vi "Push Incons.vi"(10 "node ref in":refnum<data-value>, 11 "adstar in":refnum<class "NI_Robotics_AnytimeDStar.lvclass">) -> (2 "node ref out":refnum<data-value>, 3 "adstar out":refnum<class "NI_Robotics_AnytimeDStar.lvclass">)   [LabVIEW 2017, in "NI_Robotics_AnytimeDStar.lvclass"]
uses:
  <vilib>/robotics/Navigation/Anytime D Star/NI_Robotics_AnytimeDStar.lvclass
  <vilib>/robotics/Navigation/shared/MapNode/AbstractDstarNode/NI_Robotics_AbstractDstarNode.lvclass
  <vilib>/robotics/Navigation/Anytime D Star/NI_Robotics_AnytimeDStar.lvclass/NI_Robotics_AnytimeDStar.ctl
  <vilib>/robotics/Navigation/shared/InconsistentList/NI_Robotics_InconsistentList.lvclass
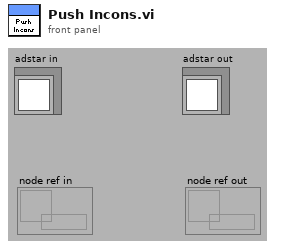
[diagram p1: front panel]
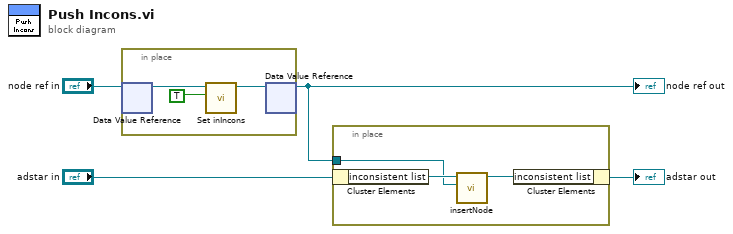
[diagram p0: block diagram]
diagram:
  n1 = in-place {
    n2 = in-place-dvr #1("node ref in") -> (w7:refnum<class "NI_Robotics_AbstractDstarNode.lvclass">)  [unwired: 1 out]
    n3 = call <vilib>:"Set inIncons.vi"("inIncons"=TRUE, "AbstractDstarNode in"=w7) -> ("AbstractDstarNode out"=w6:refnum<class "NI_Robotics_AbstractDstarNode.lvclass">)  [unwired: 9 in]
    n4 = in-place-dvr #1(w6) -> (w1:refnum<data-value>)  [unwired: 1 out]
  }
  "node ref out" <- w1
  n5 = in-place {
    in-place-border: w1 -> [w8]
    n6 = in-place-cluster #2("adstar in") -> ("inconsistent list"=w10:refnum<class "NI_Robotics_InconsistentList.lvclass">)
    n7 = call <vilib>:"insertNode.vi"("node ref in"=w8, "InconsistentList in"=w10) -> ("InconsistentList out"=w9:refnum<class "NI_Robotics_InconsistentList.lvclass">)  [unwired: 8 in, 1 out]
    n8 = in-place-cluster #2("inconsistent list"=w9) -> (→"adstar out":refnum<class "NI_Robotics_AnytimeDStar.lvclass">)
  }
